vi "Main.vi"() -> ()   [LabVIEW 2015]
uses:
  TypeDefs/States.ctl
  TypeDefs/Acq Loop Data.ctl
  TypeDefs/Buttons UI.ctl
panel:
  in  "#samples":dbl=100.0
  in  "Frequency":dbl=1000.0
  out "File Path":path
  in  "File Name Prefix":string="LV Academy"
  in  "Buttons":T1
  out "Wykres":dbl[](graph)
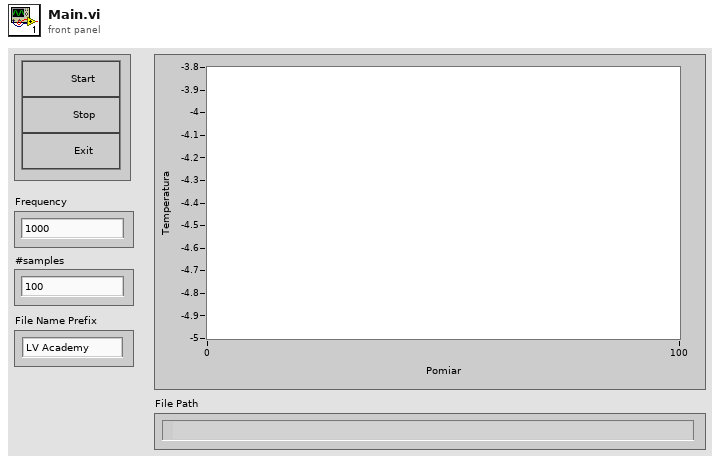
[diagram p1: front panel]
types:
  T1 = typedef "Buttons UI.ctl" = cluster{"Start":bool, "Stop":bool, "Exit":bool}
  T2 = typedef "Acq Loop Data.ctl" = cluster{"File Name Profix":string, "Frequency":dbl, "#samples":i32, "DAQ task ":refnum<k21>}
  T3 = typedef "Queue Data" = cluster{"Action":string, "Data":dbl[]}
  T4 = typedef "States.ctl" = enum16{"Check if Stop or Exit", "Exit", "Wait for Start or Exit", "Start Acquisition", "Reset Acquisition", "Acquisition"}
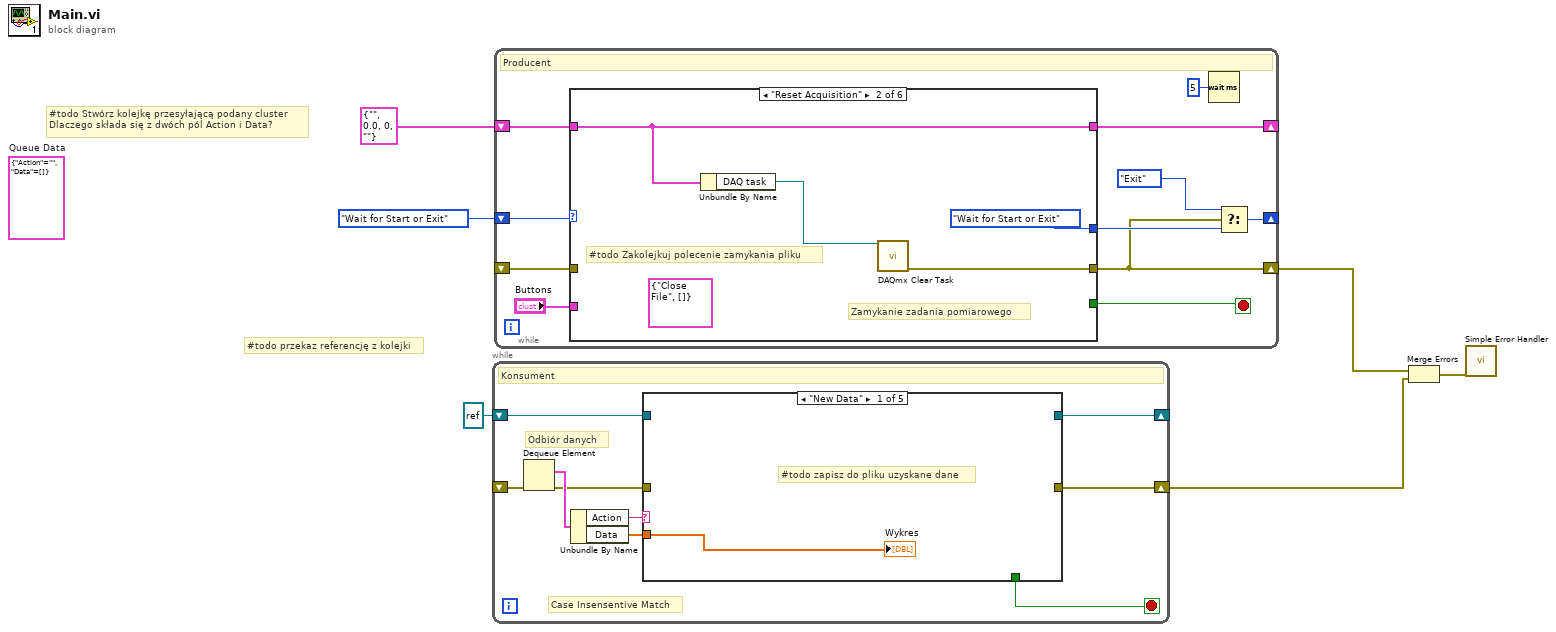
[diagram p0: block diagram]
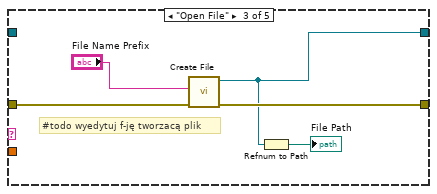
[diagram p3: hidden frame]
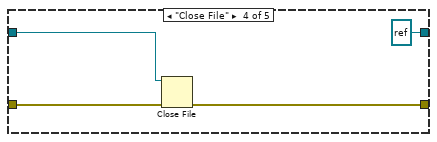
[diagram p4: hidden frame]
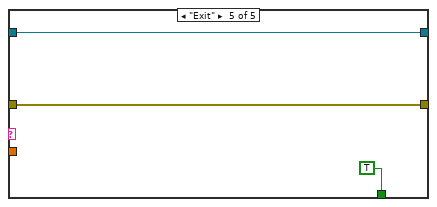
[diagram p5: hidden frame]
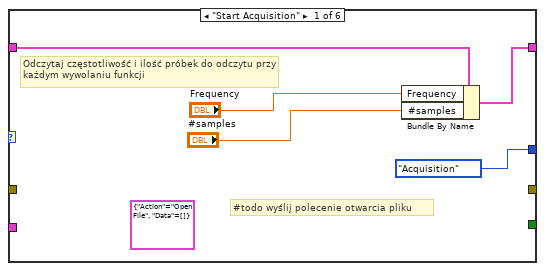
[diagram p6: hidden frame]
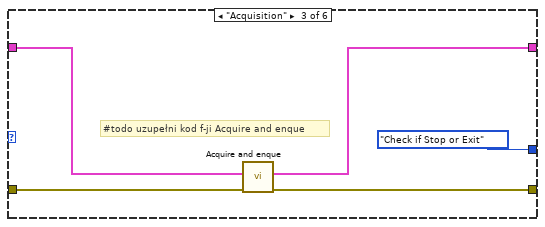
[diagram p7: hidden frame]
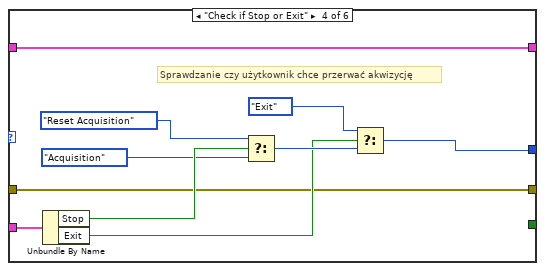
[diagram p8: hidden frame]
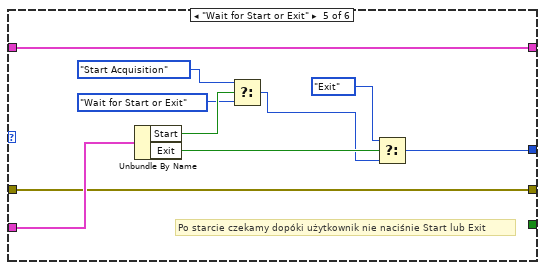
[diagram p9: hidden frame]
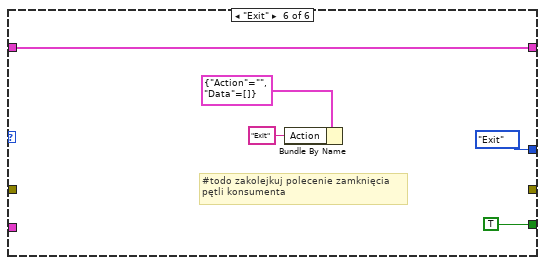
[diagram p10: hidden frame]
diagram:
  (unwired) T3 {"Action"="", "Data"=[]}  # Queue Data
  # "#todo przekaz referencję z kolejki"
  # "#todo Stwórz kolejkę przesyłającą podany cluster\nDlaczego składa się z dwóch pól Action i Data?"
  n1 = while {
    shift-right: [w9] -> w3
    shift-left: _ -> [w15]
    shift-right: [w10] -> _
    shift-left: refnum<file> refnum ("refnum out") -> [w8]
    stop <- w7 stop-if-true
    # "Odbiór danych"
    # "Case Insensentive Match"
    # "Konsument"
    n2 = Dequeue Element(error in (no error)=w15) -> (element=w14:T3, error out=w11:errorcluster)  [unwired: 2 in, 2 out]
    n3 = Unbundle By Name(w14) -> ("Action"=w13:string, "Data"=w12:dbl[])
    n4 = case shown="\"New Data\"" w13 {
      tunnel: w12 -> [w16 _ _ _ _]
      tunnel: w11 -> [_ w18 w23 w27 w29]
      tunnel: [_ w17 w19 refnum<file> refnum ("refnum out") w28] -> w10
      tunnel: [_ w18 w21 w25 w29] -> w9
      tunnel: w8 -> [_ w17 _ w26 w28]
      tunnel: [_ _ _ _ TRUE] -> w7
      frame "New Data" {
        # "#todo zapisz do pliku uzyskane dane"
        "Wykres" <- w16
      }
      frame Default {
      }
      frame "Open File" {
        # "#todo wyedytuj f-ję tworzacą plik"
        n5 = call "Create File.vi"("error in (no error)"=w23, "File Name Prefix"="File Name Prefix") -> ("error out"=w21:errorcluster, "refnum out"=w19:refnum<file>)  [unwired: 8 in]
        n6 = Refnum to Path(1:w19) -> (0:→"File Path":path)
      }
      frame "Close File" {
        n7 = Close File(refnum=w26, error in=w27) -> (error out=w25:errorcluster)  [unwired: 1 out]
      }
      frame "Exit" {
      }
    }
  }
  n8 = while {
    shift-right: [w33] -> _
    shift-left: States."Wait for Start or Exit" -> [w41]
    shift-right: [w37] -> _
    shift-left: T2 {"File Name Profix"="", "Frequency"=0.0, "#samples"=0, "DAQ task "=""} -> [w38]
    shift-right: [w31] -> w2
    shift-left: _ -> [w40]
    stop <- w35 stop-if-true
    # "Producent"
    n9 = case shown="\"Reset Acquisition\"" w41 {
      tunnel: w40 -> [_ _ w55 w57 w68 _]
      tunnel: "Buttons" -> [_ _ _ w65 w75 _]
      tunnel: [States."Acquisition" States."Wait for Start or Exit" States."Check if Stop or Exit" w58 w70 States."Exit"] -> w34
      tunnel: w38 -> [w46 w47 w54 w56 w69 w77]
      tunnel: [w43 w47 w51 w56 w69 w77] -> w37
      tunnel: [_ w50 w53 w57 w68 _] -> w31
      tunnel: [_ _ _ _ _ TRUE] -> w35
      frame "Start Acquisition" {
        (unwired) T3 {"Action"="Open File", "Data"=[]} ("element")
        # "#todo wyślij polecenie otwarcia pliku"
        # "Odczytaj częstotliwość i ilość próbek do odczytu przy każdym wywolaniu funkcji"
        n10 = Bundle By Name(cluster=w46, "Frequency"="Frequency", "#samples"="#samples") -> (w43:T2)
      }
      frame "Reset Acquisition" {
        (unwired) T3 {"Action"="Close File", "Data"=[]} ("element")
        # "#todo Zakolejkuj polecenie zamykania pliku"
        # "Zamykanie zadania pomiarowego"
        n11 = Unbundle By Name(w47) -> ("DAQ task"=w49:refnum<k21>)
        n12 = call <vilib>:"DAQmx Clear Task.vi"("task in"=w49) -> ("error out"=w50:errorcluster)  [unwired: 14 in]
      }
      frame "Acquisition" {
        # "#todo uzupełni kod f-ji Acquire and enque"
        n13 = call "Acquire and enque.vi"("error in (no error)"=w55, "Data In"=w54) -> ("error out"=w53:errorcluster, "Data Out"=w51:T2)  [unwired: 8 in]
      }
      frame "Check if Stop or Exit" {
        # "Sprawdzanie czy użytkownik chce przerwać akwizycję"
        n14 = Unbundle By Name(w65) -> ("Stop"=w64:bool, "Exit"=w60:bool)
        n15 = Select(t=States."Reset Acquisition", s=w64, f=States."Acquisition") -> (s? t:f=w61:T4)
        n16 = Select(t=States."Exit", s=w60, f=w61) -> (s? t:f=w58:T4)
      }
      frame "Wait for Start or Exit" {
        # "Po starcie czekamy dopóki użytkownik nie naciśnie Start lub Exit"
        n17 = Unbundle By Name(w75) -> ("Start"=w74:bool, "Exit"=w71:bool)
        n18 = Select(t=States."Start Acquisition", s=w74, f=States."Wait for Start or Exit") -> (s? t:f=w67:T4)
        n19 = Select(t=States."Exit", s=w71, f=w67) -> (s? t:f=w70:T4)
      }
      frame "Exit" {
        # "#todo zakolejkuj polecenie zamknięcia\npętli konsumenta"
        n20 = Bundle By Name(cluster=T3 {"Action"="", "Data"=[]}, "Action"="Exit") -> ()  [unwired: 1 out]
      }
    }
    n21 = Wait (ms)(milliseconds to wait=u32 5) -> ()  [unwired: 1 out]
    n22 = Select(t=States."Exit", s=w31, f=w34) -> (s? t:f=w33:T4)
  }
  n23 = Merge Errors(w2, w3) -> (w1:errorcluster)
  n24 = call <vilib>:"Simple Error Handler.vi"("error in (no error)"=w1) -> ()  [unwired: 4 in, 5 out]
